vi "Serialize Data.vi"(8 "error in (no error)":errorcluster, 11 "Process Data":T1={"Timestamp"=0, "Antenna Connected"=FALSE, "Satellites"=0, "Mobile Mode"=FALSE, "Location"={"Latitude"=0.0, "Longitude"=0.0, "Altitude"=0.0}, "Velocity"={"East"=0.0, "North"=0.0, "Up"=0.0}, "GPS state"=11, "UTC Offset"=0, "UTC Offset Valid"=FALSE} {"GPS state" items=["Uninitialized", "Antenna Error", "No Useable Satellites", "One Useable Satellite", "Two Useable Satellites", "Three Useable Satellites", "No GPS Time", "PDOP Too High", "Unusable Satellite", "Fix Rejected", "Self Survey Complete", "Self Survey Not Complete"]}) -> (0 "error out":errorcluster, 3 "Flat Data out":string)   [LabVIEW 2020, in "GPS.lvlib"]
doc: "Version 0.1"
uses:
  <vilib>/ADAS Record/CustomDataTypes/GPS/GPS.lvlib
  <vilib>/ADAS Record/CustomDataTypes/GPS/Process Data.ctl
  <vilib>/ADAS Record/IODataPEF/CfgMgr/FlatFormat.ctl
  69b4f655-d322-486f-8d65-ee31f7d8c6ef.vi
  <vilib>/ADAS Record/IODataPEF/Error/Error_CheckAndSetDllError.vi
  <vilib>/ADAS Record/IODataPEF/Error/Error_SetError.vi
  <vilib>/ADAS Record/IODataPEF/CfgMgr/GetPEFConfiguration_DefaultFlatFormat.vi
  <vilib>/ADAS Record/IODataPEF/Error/ErrorMgr.vi
  <vilib>/ADAS Record/CustomData/_Custom_RegisterType.vi
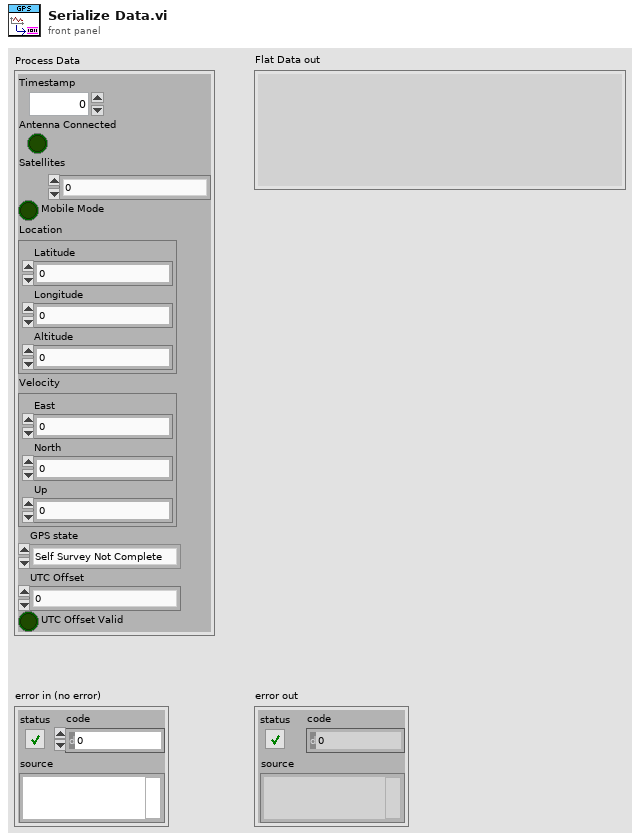
[diagram p1: front panel]
types:
  T1 = typedef "GPS.lvlib/Process Data.ctl" = cluster{"Timestamp":u64, "Antenna Connected":bool, "Satellites":u32, "Mobile Mode":bool, "Location":cluster{"Latitude":dbl, "Longitude":dbl, "Altitude":dbl}, "Velocity":cluster{"East":dbl, "North":dbl, "Up":dbl}, "GPS state":u32, "UTC Offset":i32, "UTC Offset Valid":bool}
  T2 = typedef "FlatFormat.ctl" = enum32{"Auto", "PEF", "GFB (Apache)", "GFB", "JSON", "Readable JSON", "LV String", "Reserved", "LV Native"}
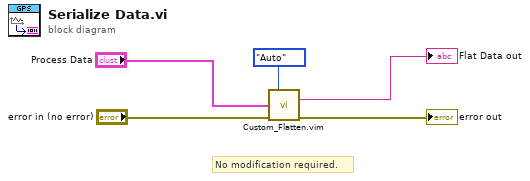
[diagram p0: block diagram]
diagram:
  # "No modification required."
  n1 = call "Custom_Flatten.vim"("Flat Format"=FlatFormat."Auto", "Data"="Process Data", "error in (no error)"="error in (no error)") -> ("Flat Data"=→"Flat Data out":string, "Error (out)"=→"error out":errorcluster)  [unwired: 10 in, 1 out]
